vi "VNA Empty Driver Input.vi"() -> (0 "VNA Driver Input":T1={"VNA Command"=enum."MEASURE", "VNA Driver or\nVNA Configuration (\"\")"="", "Parameters to Measure"=[], "VNA Stimulus"={"Use Instrument Settings"=FALSE, "Blank Frequencies"=FALSE, "Sweep Type"=enum."Linear", "Sweep"={"Fstart"=500.0, "Fstop"=1500.0, "Units"=enum."MHz", "Points"=201}, "Power (dBm)"=999.0, "IFBW (Hz)"=-1.0, "Sweep Time (s)"=-1.0, "Calibration"={"State"=FALSE, "String"=""}}, "Miscellaneous Parameters"={"Formatted Data"=FALSE, "Auto Select"=FALSE, "Seq Count"=0}, "Drv Refnum"=refnum} {"Parameters to Measure"."Channel" min=1 max=99 step=1; "Parameters to Measure"."Parameter"."Stimulus Port" min=1 step=1; "Parameters to Measure"."Parameter"."Response Port" min=1 step=1; "VNA Stimulus"."Sweep Time (s)" format="%.3g"})   [LabVIEW 2011]
uses:
  tests/S Parameter/TypeDefs/SP Frequency Units.ctl
  tests/S Parameter/TypeDefs/SP Stimulus Parameters.ctl
  tests/S Parameter/TypeDefs/SP Parameter.ctl
  tests/S Parameter/TypeDefs/SP Calibration State.ctl
  VNA Measurement Format.ctl
  VNA Parameter to Measure.ctl
  VNA Command.ctl
  VNA Driver Ref.ctl
  tests/S Parameter/TypeDefs/SP Miscellaneous Parameters.ctl
  VNA Driver Input.ctl
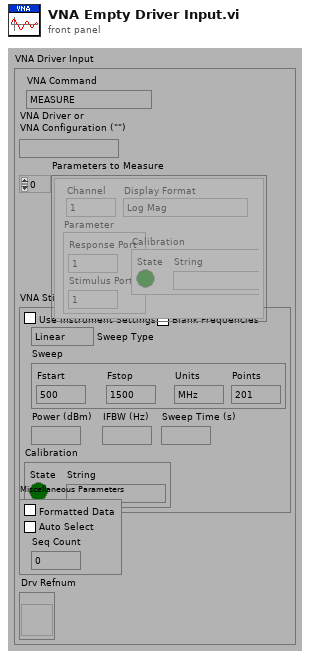
[diagram p1: front panel]
types:
  T1 = typedef "VNA Driver Input.ctl" = cluster{"VNA Command":T2, "VNA Driver or\nVNA Configuration (\"\")":string, "Parameters to Measure":T3[], "VNA Stimulus":T7, "Miscellaneous Parameters":T9, "Drv Refnum":T10}
  T2 = typedef "VNA Command.ctl" = enum16{"LOAD", "INITIALIZE", "PRESET", "GET STIMULUS", "SET STIMULUS", "GET CALIBRATION", "CALIBRATE", "RESTORE", "MEASURE", "RELEASE", "UNLOAD", "CONFIRM", "SORT"}
  T3 = typedef "VNA Parameter to Measure.ctl" = cluster{"Channel":i8, "Parameter":T4, "Calibration":T5, "Display Format":T6}
  T4 = typedef "SP Parameter.ctl" = cluster{"Stimulus Port":i8, "Response Port":i8}
  T5 = typedef "SP Calibration State.ctl" = cluster{"State":bool, "String":string}
  T6 = typedef "VNA Measurement Format.ctl" = enum32{"Log Mag", "Phase", "Delay", "Smith (R+jX)", "Polar (Re/Im)", "Linear Mag", "SWR", "Real", "Imaginary", "Smith (Lin/Phase)", "Smith (Log/Phase)", "Smith (Real/Imag)", "Smith (G+jB)", "Polar (Lin)", "Polar (Log)", "Expanded Phase", "Positive Phase", "Inverted Smith", "Unwrapped Phase", "Power Out"}
  T7 = typedef "SP Stimulus Parameters.ctl" = cluster{"Use Instrument Settings":bool, "Blank Frequencies":bool, "Sweep Type":enum32{"Linear", "Logarithmic", "List", "Power", "CW"}, "Sweep":cluster{"Fstart":dbl, "Fstop":dbl, "Units":T8, "Points":i32}, "Power (dBm)":dbl, "IFBW (Hz)":dbl, "Sweep Time (s)":dbl, "Calibration":T5}
  T8 = typedef "SP Frequency Units.ctl" = enum16{"Hz", "kHz", "MHz", "GHz", "Points"}
  T9 = typedef "SP Miscellaneous Parameters.ctl" = cluster{"Formatted Data":bool, "Auto Select":bool, "Seq Count":u32}
  T10 = typedef "VNA Driver Ref.ctl" = refnum<vi>
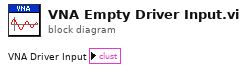
[diagram p0: block diagram]
diagram:
